vi "Configure VIP Uninstall.vi"(8 "error in (no error)":errorcluster, 10 "JSON string":string) -> (0 "error out":errorcluster, 3 "VIP Install Out":refnum<class "VIP Uninstall.lvclass">)   [LabVIEW 2014, in "VIP Uninstall.lvclass"]
uses:
  VIP Uninstall.lvclass
  VIP Uninstall - STYP.ctl
  VIP Uninstall.lvclass/VIP Uninstall.ctl
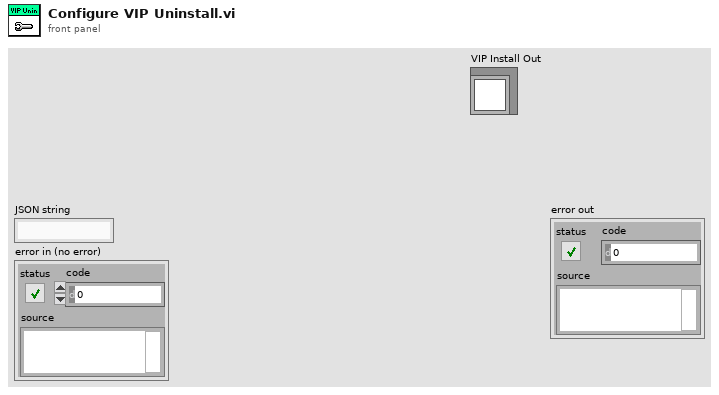
[diagram p1: front panel]
types:
  T1 = typedef "VIP Uninstall - STYP.ctl" = cluster{"VIP Name":string, "LabVIEW Version":string}
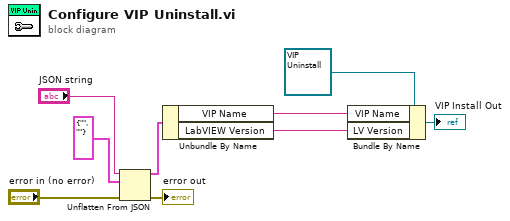
[diagram p0: block diagram]
diagram:
  n1 = Unflatten From JSON(JSON string="JSON string", type and defaults=T1 {"VIP Name"="", "LabVIEW Version"=""} ("VIP Publish"), error in (no error)="error in (no error)") -> (value=w5:T1, error out=→"error out":errorcluster)  [unwired: 4 in]
  n2 = Unbundle By Name(w5) -> ("VIP Name"=w3:string, "LabVIEW Version"=w2:string)
  n3 = Bundle By Name(cluster=refnum<class "VIP Uninstall.lvclass"> refnum ("VIPB Build out"), "VIP Name"=w3, "LV Version"=w2) -> (→"VIP Install Out":refnum<class "VIP Uninstall.lvclass">)
